vi "Set Output.vi"(8 "error in (no error)":errorcluster, 10 "Enable?":bool, 11 "Keysight in":refnum<class "PS Keysight.lvclass">) -> (0 "error out":errorcluster, 3 "Keysight out":refnum<class "PS Keysight.lvclass">)   [LabVIEW 2021, in "PS.lvlib" / "PS Keysight.lvclass"]
uses:
  PS Keysight.lvclass
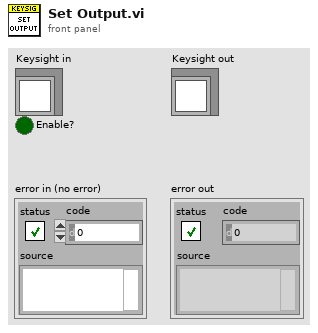
[diagram p1: front panel]
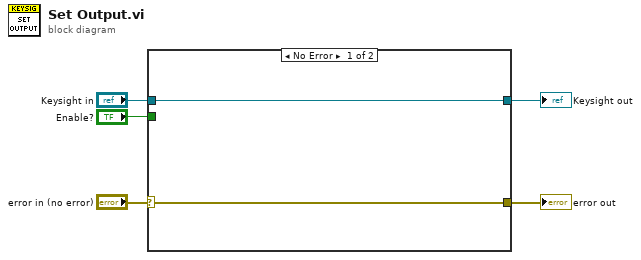
[diagram p0: block diagram]
diagram:
  n1 = case shown="No Error" "error in (no error)" {
    selector: "error in (no error)" -> [w6 w8]
    tunnel: [w7 w9] -> w4
    tunnel: "Keysight in" -> [w7 w9]
    tunnel: [w6 w8] -> w2
    tunnel: "Enable?" -> [_ _]
    frame No Error {
    }
    frame Error {
    }
  }
  "error out" <- w2
  "Keysight out" <- w4
